vi "Read Build Trigger.vi"(8 "error in (no error)":errorcluster, 11 "Job Initialize in":refnum<class "Job Initialize.lvclass">) -> (0 "error out":errorcluster, 2 "Cron":T1={"Day of Week"=enum."Everyday", "Hour"=1, "Enable?"=FALSE} {"Hour" min=0 max=23}, 3 "Job Initialize out":refnum<class "Job Initialize.lvclass">)   [LabVIEW 2014, in "Job Initialize.lvclass"]
uses:
  Job Initialize.lvclass
  Controls/Cron String - STYP.ctl
  Job Initialize.lvclass/Job Initialize.ctl
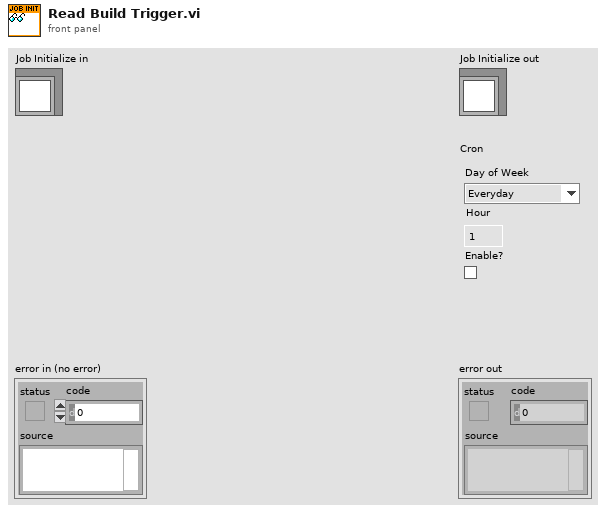
[diagram p1: front panel]
types:
  T1 = typedef "Cron String - STYP.ctl" = cluster{"Day of Week":enum16{"Everyday", "Sunday", "Monday", "Tuesday", "Wednesday", "Thursday", "Friday", "Saturday"}, "Hour":i32, "Enable?":bool}
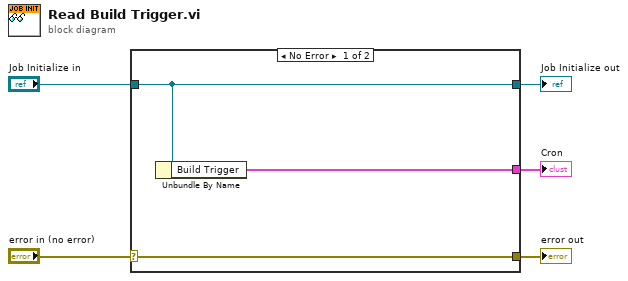
[diagram p0: block diagram]
diagram:
  n1 = case shown="No Error" "error in (no error)" {
    selector: "error in (no error)" -> [w8 w9]
    tunnel: [w8 w9] -> w4
    tunnel: [w7 w10] -> w2
    tunnel: "Job Initialize in" -> [w7 w10]
    tunnel: [w6 _] -> w1
    frame No Error {
      n2 = Unbundle By Name(w7) -> ("Build Trigger"=w6:T1)
    }
    frame Error {
    }
  }
  "error out" <- w4
  "Job Initialize out" <- w2
  "Cron" <- w1
